vi "Digital input.vi"(8 "error in":errorcluster, 9 "test input":bool, 10 "test":bool, 11 "task/channels in":refnum<k21>) -> (0 "error out":errorcluster, 3 "element 2":bool)   [LabVIEW 2013]
uses:
  <vilib>/DAQmx/read.llb/DAQmx Read.vi
  <vilib>/DAQmx/read.llb/DAQmx Read (Digital 1D Bool NChan 1Samp 1Line).vi
  <vilib>/DAQmx/miscellaneous.llb/DAQmx Fill In Error Info.vi
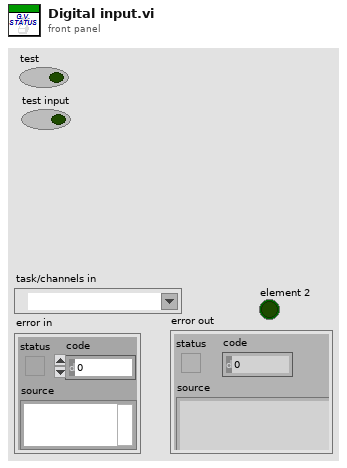
[diagram p1: front panel]
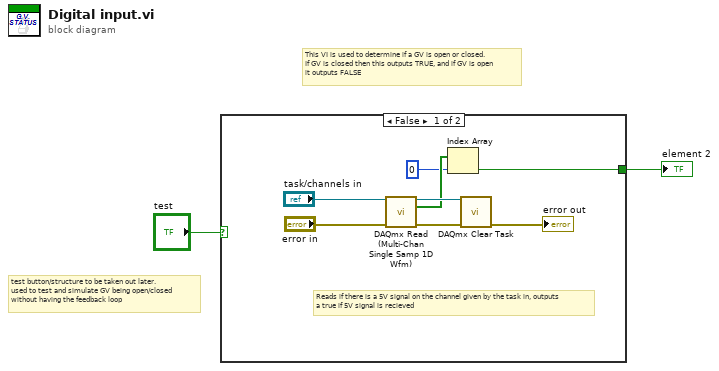
[diagram p0: block diagram]
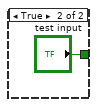
[diagram p2: hidden frame]
diagram:
  # "This VI is used to determine if a GV is open or closed. \nIf GV is closed then this outputs TRUE, and if GV is open\nit outputs FALSE"
  # "test button/structure to be taken out later.\nused to test and simulate GV being open/closed\nwithout having the feedback loop"
  n1 = case shown="False" "test" {
    tunnel: [w3 "test input"] -> w1
    frame False {
      # "Reads if there is a 5V signal on the channel given by the task in, outputs\na true if 5V signal is recieved"
      n2 = call-poly "DAQmx Read (Multi-Chan Single Samp 1D Wfm).vi"("task/channels in"="task/channels in", "error in"="error in") -> ("task out"=w9:refnum<k21>, "data"=w6:bool[], "error out"=w10:errorcluster)  [unwired: 11 in]
      n3 = Index Array(array=w6, index=0) -> (element=w3:bool)
      n4 = call <vilib>:"DAQmx Clear Task.vi"("task in"=w9, "error in"=w10) -> ("error out"=→"error out":errorcluster)  [unwired: 13 in]
    }
    frame True {
    }
  }
  "element 2" <- w1
